vi "lab1.vi"() -> ()   [LabVIEW 2020]
panel:
  out "Array 5":i16[][](array[numeric])
  out "Array 4":i16[][](array[numeric])
  out "Array 3":i16[][](array[numeric])
  in  "Array str":dbl
  in  "Array col":dbl
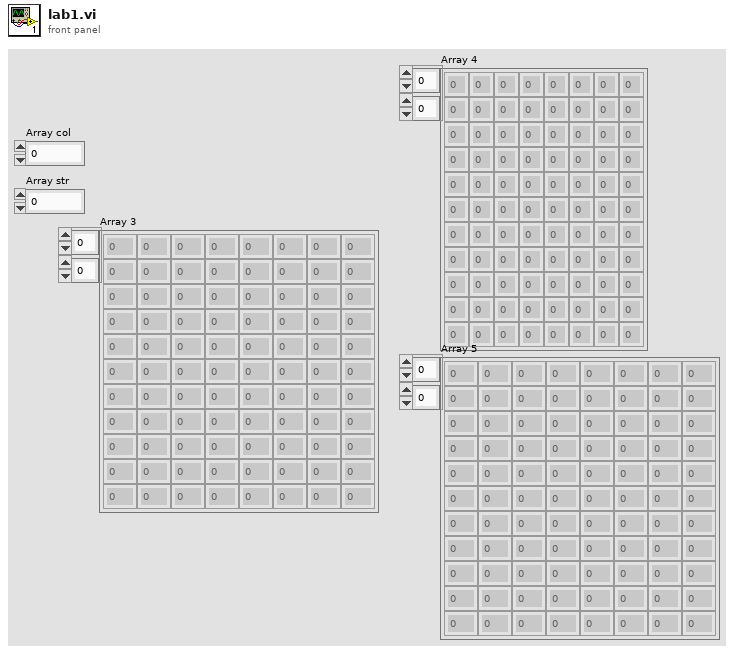
[diagram p1: front panel]
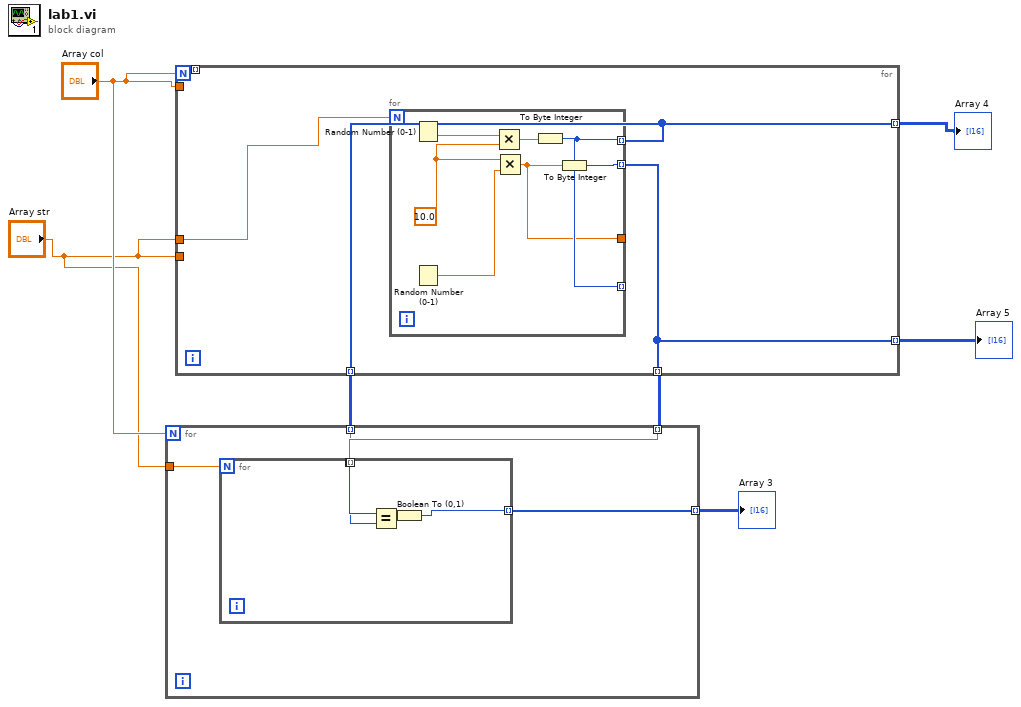
[diagram p0: block diagram]
diagram:
  n1 = for {
    N: "Array col" -> [w11]
    tunnel: [w11] -> _ mode=indexing
    tunnel: [w9] -> w2 mode=indexing
    tunnel: [w8] -> w4 mode=indexing
    tunnel: "Array str" -> [w10]
    tunnel: "Array col" -> [_]
    tunnel: "Array str" -> [_]
    tunnel: [w9] -> w3 mode=indexing
    tunnel: [w8] -> w1 mode=indexing
    n2 = for {
      N: w10 -> [_]
      tunnel: [w12] -> w8 mode=indexing
      tunnel: [w14] -> w9 mode=indexing
      tunnel: [w13] -> _
      tunnel: [w14] -> _ mode=indexing
      w17 = 10.0 ("y")
      n3 = Random Number (0-1)() -> (number: 0 to 1=w18:dbl)
      n4 = Random Number (0-1)() -> (number: 0 to 1=w16:dbl)
      n5 = Multiply(x=w18, y=w17) -> (x*y=w15:dbl)
      n6 = Multiply(x=w17, y=w16) -> (x*y=w13:dbl)
      n7 = To Byte Integer(number=w15) -> (8bit integer=w14:i8)
      n8 = To Byte Integer(number=w13) -> (8bit integer=w12:i8)
    }
  }
  "Array 4" <- w2
  "Array 5" <- w1
  n9 = for {
    N: "Array col" -> [_]
    tunnel: "Array str" -> [w22]
    tunnel: [w21] -> w7 mode=indexing
    tunnel: w4 -> [w20] mode=indexing
    tunnel: w3 -> [w19] mode=indexing
    n10 = for {
      N: w22 -> [_]
      tunnel: [w25] -> w21 mode=indexing
      tunnel: w20 -> [w24] mode=indexing
      tunnel: w19 -> [w23] mode=indexing
      n11 = Equal?(x=w24, y=w23) -> (x = y?=w26:bool)
      n12 = Boolean To (0,1)(Boolean=w26) -> (0, 1=w25:i16)
    }
  }
  "Array 3" <- w7
